vi "nanocal -- generate 3D curvature ellipsoid --  V4.vi"(6 "sampling vicinity size (%)":dbl, 7 "error mode":T7=enum."errors-linear", 8 "newton parameters":T9={"newton action"=enum."onlygrads", "weighting"=enum."dω √(|dz/dω|)", "PID-P"=0.009761510697263134, "PID-I"=5} {"PID-P" scale=1e-09..1.0 scale format="%#_3p"}, 9 "data":T8={"dz/dω  (sec/rad)"=[], "z "=[1.7183506006211996e-05-0.0001154032788780638i, 1.7124360968751133e-05-0.0001154114779288915i, 1.7049104347380084e-05-0.00011541542942613611i, 1.700437896335042e-05-0.00011541749156201827i, 1.6984579723285106e-05-0.00011542204741013496i, 1.702277369054923e-05-0.00011543195548892015i, 1.713094025845651e-05-0.00011543928112855599i, 1.734249707866828e-05-0.00011543960094139092i, 1.768320429215342e-05-0.0001154245402225022i, 1.8195281152538477e-05-0.00011538335923575508i, 1.8917228661806973e-05-0.00011530288392402138i, 1.9897834564883332e-05-0.00011516640933089982i, 2.154104046962704e-05-0.0001148906117047364i, 2.3247799321765792e-05-0.00011455940834964969i, 2.5364678450551808e-05-0.00011410149936074356i, 2.8645788781885885e-05-0.00011331572480450341i, 3.204749554800641e-05-0.00011242961468546203i, 3.783559691555022e-05-0.00011080033368711338i, 4.245015867332296e-05-0.00010941815048749576i, 4.909131821431355e-05-0.0001073312840925185i, 5.511821898441184e-05-0.00010535829212367013i, 6.178843506022867e-05-0.00010310289174359778i, 7.1079604965352e-05-9.985157907779013e-05i, 7.922304381453334e-05-9.690255343156676e-05i, 8.814778883893872e-05-9.35627973091444e-05i, 9.806709148886077e-05-8.971246458508318e-05i, 0.00011119043245647465-8.437841897470898e-05i, 0.00012253184919712196-7.953180105990741e-05i, 0.00013777724317049346-7.26422052575784e-05i, 0.0001508081004573332-6.638511645494567e-05i, 0.00016547294918783876-5.890291826790314e-05i, 0.00018003847596605868-5.097295421607585e-05i, 0.00019518361086534857-4.2160672625888326e-05i, 0.00021134179818259658-3.207632261667366e-05i, 0.0002372041782935464-1.434566976209705e-05i, 0.00025518143132024254-7.65423157605567e-07i, 0.0002835129702467886+2.297908707067173e-05i, 0.0003060118087631287+4.414715126576145e-05i, 0.00032860772064336976+6.780161699354136e-05i, 0.0003492674091322389+9.188627597766353e-05i, 0.00037498324855458583+0.0001258445655672888i, 0.00040021078021115026+0.00016463936720210011i, 0.00041969942568205823+0.0001996255883353531i, 0.00044367338947118773+0.00025154867300893595i, 0.0004634793607238068+0.0003068834938295352i, 0.00047921028781215815+0.00036805191402776324i, 0.0004880906353641744+0.00042166295770603194i, 0.0004932212623741357+0.0004947057496862386i, 0.000491476456593048+0.0005562791342814882i, 0.000480893803992059+0.0006363872629062725i, 0.0004535995818650303+0.0007373086546111893i, 0.000417087772881063+0.0008226852134031236i, 0.0003564148692854789+0.0009214817173403453i, 0.0003049201646356487+0.0009841224100520793i, 0.00021260191240459413+0.0010684135492785532i, 0.00011714858948470126+0.001130293664798013i, 1.675457544365132e-05+0.0011752384955043165i, -6.8674075405897e-05+0.0012001399159748158i, -0.000156473047607305+0.0012143601357779102i, -0.00026709373934749337+0.0012167952520739987i, -0.0003544271565676041+0.001206585218500233i, -0.00047937600197311275+0.0011721904461218277i, -0.0006086290582260493+0.0011080263068835828i, -0.0007031877411848573+0.0010369948237613604i, -0.0007564526901441745+0.0009845652865779295i, -0.000802489180995596+0.0009292050493656664i, -0.0008414596018105983+0.0008721985101652608i, -0.0008809346482248761+0.0008000538120167723i, -0.0009073902840241921+0.0007382113118499092i, -0.0009264953054508651+0.000680980624166274i, -0.0009405659412141811+0.0006247883223244968i, -0.000951649722530156+0.0005564170049287236i, -0.0009557485581057351+0.0005027508202624884i, -0.0009558464741053665+0.0004515634249715623i, -0.0009509110176922098+0.0003899637122391104i, -0.0009411315169847015+0.00033238768338539245i, -0.0009303400913929496+0.0002890952314710416i, -0.0009171113529290538+0.00024772942260094455i, -0.0009022111527275027+0.00020961974320628598i, -0.0008813746494947608+0.00016554205395646727i, -0.0008581837971946129+0.00012481593212717478i, -0.0008372063466683705+9.328565348151487e-05i, -0.0008165626610594428+6.595676342721183e-05i, -0.0007901155435838691+3.51376371228606e-05i, -0.0007682834352800848+1.2585785624721776e-05i, -0.000746231015527196-7.956667433689733e-06i, -0.0007238798463130141-2.6771164006128246e-05i, -0.0007015567569177018-4.3779400880525094e-05i, -0.000679301954671598-5.9154880569231366e-05i, -0.0006572001413831251-7.301304884663801e-05i, -0.000629855254567978-8.838260380910578e-05i, -0.0006083942229188815-9.917719243438264e-05i, -0.0005768631156754208-0.00011317657292622015i, -0.0005562177438951648-0.00012121832857134644i, -0.0005359092039599222-0.00012831021292074535i, -0.0005145186443378148-0.00013494179211461784i, -0.0004951602053444319-0.00014023403510992087i, -0.00047624970229075174-0.00014478034103386663i, -0.0004577401041527736-0.00014865456703421655i, -0.00043519037796120065-0.00015262867452433312i], "ω (rad/sec)"=[32012.991918577427, 32390.261658505893, 32466.39798177853, 32499.14340521798, 32517.39286113775, 32529.046092051318, 32537.14525712326, 32543.111142615544, 32547.696343954158, 32551.33675949651, 32554.302325209504, 32556.769142360055, 32558.856995237307, 32560.650202739795, 32562.209843476354, 32563.58125099723, 32564.7987833122, 32565.88895894197, 32566.872575330308, 32567.766175404246, 32568.583086316496, 32569.334166794306, 32570.02835688638, 32570.673085530187, 32571.274580490695, 32571.838104118455, 32572.36813539066, 32572.868514009202, 32573.342552524307, 32573.793126289274, 32574.222746575288, 32574.633618125405, 32575.027687968828, 32575.40668442971, 32575.772149741057, 32576.12546690325, 32576.467883345118, 32576.800529469096, 32577.124435064776, 32577.440543590797, 32577.749724325146, 32578.052781957467, 32578.35046682089, 32578.643482565894, 32578.932492128843, 32579.218126471686, 32579.500987779396, 32579.781656707495, 32580.06069600583, 32580.338656060805, 32580.616078519142, 32580.89350097748, 32581.171461032456, 32581.45050033079, 32581.73116925889, 32582.0140305666, 32582.29966469628, 32582.58867447239, 32582.88169000423, 32583.179375080817, 32583.48243271314, 32583.791613234323, 32584.10772197351, 32584.43162756919, 32584.764273480003, 32585.106690135035, 32585.460007297228, 32585.825472395412, 32586.204468856296, 32586.59853891288, 32587.009410462997, 32587.439030535847, 32587.889604513977, 32588.363642815923, 32588.86402143446, 32589.39405291983, 32589.957576334426, 32590.559071508098, 32591.203800151903, 32591.897990030815, 32592.64907072179, 32593.46598163404, 32594.359581707977, 32595.343197883154, 32596.433373726086, 32597.650906041054, 32599.022313348767, 32600.58195429849, 32602.375161800977, 32604.46301467823, 32606.929831615616, 32609.895397541775, 32613.535812870963, 32618.12101442274, 32624.086899701866, 32632.186064986967, 32643.839295900536, 32662.088751820305, 32694.834175046595, 32770.97049853239]}, 10 "Curvature triplet array IN":T2[](array[typedef])=[{"one"=enum."τ1", "two"=enum."στ1", "sigmaone"=enum."στ1", "sigmatwo"=enum."στ1", "3D curvature"={"curvature Matrix"=[[3.0, 1.0], [1.0, 4.0]], "eigenvs"=[4.618033988749895, 2.381966011250105], "Eigenvectors"=[[-0.8506508083520399+0.0i, -0.5257311121191335+0.0i], [0.5257311121191335+0.0i, -0.8506508083520399+0.0i]], "theta (rad)"=0.5535743588970453, "theta (deg)"=31.717474411461012, "Δs"=[4.618033988749895, 2.381966011250105], "δG/G"=0.5535743588970453, "Δlog(s)"=[4.618033988749895, 2.381966011250105], "inverse Matrix"=[[3.0, 1.0], [1.0, 4.0]], "noise T"=0.5535743588970453}, "three"=enum."στ1", "sigmathree"=enum."τ1", "pars & errors"={}}] {"3D curvature"."noise T" format="%#_3f"; "3D curvature"."inverse Matrix" format="%#_3p"; "3D curvature"."Δlog(s)" scale=0.001..10.0; "3D curvature"."δG/G" format="%#_3f"; "3D curvature"."Δs" format="%#_2p"; "3D curvature"."theta (deg)" format="%#_3p"; "3D curvature"."curvature Matrix" format="%#_3p"; "3D curvature"."eigenvs" format="%#_2f"; "3D curvature"."Eigenvectors" format="%#_3p"; "3D curvature"."theta (rad)" format="%#_3p"}, 11 "parameter map":map{T3, dbl}(c390)) -> (2 "Curvature triplet array OUT":T2[](array[typedef])=[{"one"=enum."τ1", "two"=enum."στ1", "sigmaone"=enum."στ1", "sigmatwo"=enum."στ1", "3D curvature"={"curvature Matrix"=[[3.0, 1.0], [1.0, 4.0]], "eigenvs"=[4.618033988749895, 2.381966011250105], "Eigenvectors"=[[-0.8506508083520399+0.0i, -0.5257311121191335+0.0i], [0.5257311121191335+0.0i, -0.8506508083520399+0.0i]], "theta (rad)"=0.5535743588970453, "theta (deg)"=31.717474411461012, "Δs"=[4.618033988749895, 2.381966011250105], "δG/G"=0.5535743588970453, "Δlog(s)"=[4.618033988749895, 2.381966011250105], "inverse Matrix"=[[3.0, 1.0], [1.0, 4.0]], "noise T"=0.5535743588970453}, "three"=enum."στ1", "sigmathree"=enum."τ1", "pars & errors"={}}] {"3D curvature"."noise T" format="%#_3f"; "3D curvature"."inverse Matrix" format="%#_3p"; "3D curvature"."Δlog(s)" scale=0.001..10.0; "3D curvature"."δG/G" format="%#_3f"; "3D curvature"."Δs" format="%#_2p"; "3D curvature"."theta (deg)" format="%#_3p"; "3D curvature"."curvature Matrix" format="%#_3p"; "3D curvature"."eigenvs" format="%#_2f"; "3D curvature"."Eigenvectors" format="%#_3p"; "3D curvature"."theta (rad)" format="%#_3p"})   [LabVIEW 2021]
uses:
  3-lorentzian-parameters.ctl
  nanocal -- gradient descent -- parameters.ctl
  3-lorentzian-heat-response action.ctl
  nanocal-goodness-weighting-strategy.ctl
  nanocal -- gradient descent-- data.ctl
  nanocal generate curvature ellipse -- action.ctl
  3D curvature triplet control.ctl
  3D curvature tensor.ctl
  <vilib>/Analysis/Matrix/Datatypes/RealMatrix.ctl
  <vilib>/Analysis/Matrix/Datatypes/ComplexMatrix.ctl
  3-vec.ctl
  4-vec-array.ctl
  nanocal -- gradient descent -- action.ctl
  <vilib>/Analysis/baseanly.llb/Mean (DBL).vi
  3D curvature tensor algebra --V2.vi
  array -- bilinear regression 3D -- V3.vi
  <vilib>/Analysis/7linalg.llb/Solve Linear Equations.vi
  <vilib>/Analysis/7linalg.llb/Solve Linear Equations (single right hand).vi
  array -- linear regression 3D -- V2.vi
  <vilib>/Analysis/baseanly.llb/A x B.vi
  <vilib>/Analysis/baseanly.llb/Real A x B.vi
  <vilib>/Analysis/baseanly.llb/Solve Linear Equations By Cholesky.vi
  <vilib>/Analysis/baseanly.llb/Real Matrix to Compact Array.vi
  <vilib>/Analysis/baseanly.llb/Real Compact Tri-Matrix Linear Eqs.vi
  <vilib>/Analysis/Matrix/Numeric/Conversions/Array To Matrix.vi
  <vilib>/Analysis/Matrix/Numeric/Conversions/Array To Matrix - RA2.vi
  <vilib>/Analysis/7linalg.llb/Solve Linear Eqs (General).vi
  <vilib>/Analysis/7linalg.llb/Solve Linear Eqs (Gen, single right hand).vi
  <vilib>/Analysis/Matrix/Numeric/Conversions/Matrix To Array.vi
  <vilib>/Analysis/Matrix/Numeric/Conversions/Matrix To Array - RM.vi
  <vilib>/Analysis/7linalg.llb/Eigenvalues and Vectors.vi
  <vilib>/Analysis/7linalg.llb/Real Eigenvalues and Vectors.vi
  <vilib>/Analysis/baseanly.llb/Inverse Matrix.vi
  <vilib>/Analysis/baseanly.llb/Real Inverse Matrix.vi
  <vilib>/Analysis/NI_AALBase.lvlib
  <vilib>/Analysis/Matrix/NI_Matrix.lvlib
panel:
  in  "means":T1
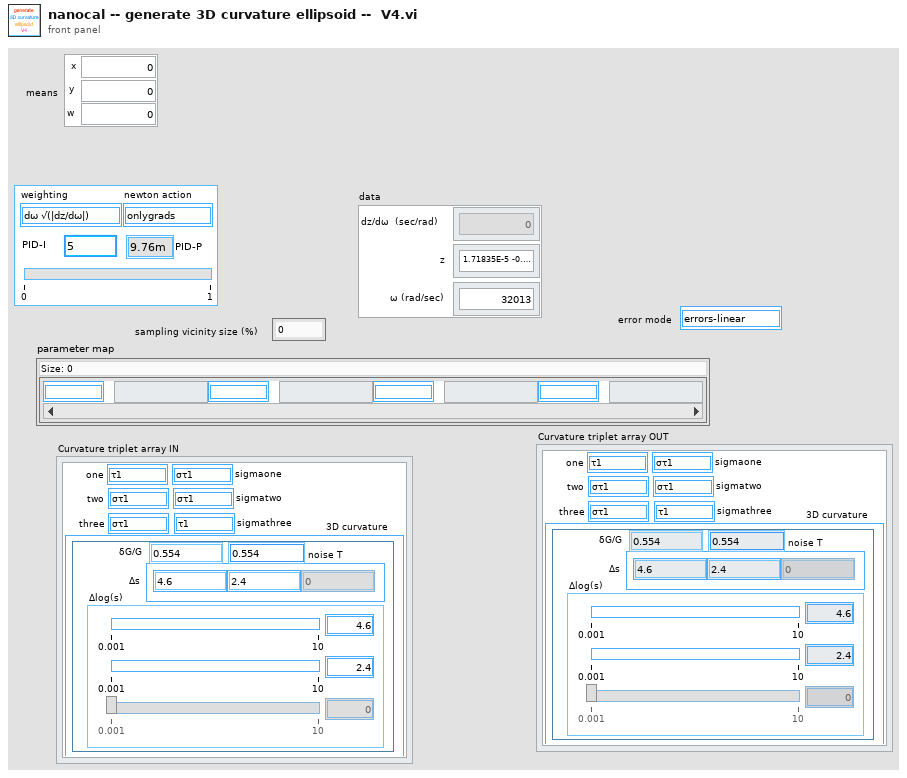
[diagram p1: front panel]
types:
  T1 = typedef "3-vec.ctl" = cluster{"x":dbl, "y":dbl, "w":dbl}
  T2 = typedef "3D curvature triplet control.ctl" = cluster{"one":T3, "two":T3, "sigmaone":T3, "sigmatwo":T3, "3D curvature":T4, "three":T3, "sigmathree":T3, "pars & errors":map{T3, dbl}}
  T3 = typedef "3-lorentzian-parameters.ctl" = enum16{"ζ", "τ1", "τS", "τN", "τC", "κ0", "m1", "m2", "m3", "T (K)", "B (T)", "θ (deg)", "side (S|R)", "set of (B|T)", "Re(offset)", "Im(offset)", "στ1", "στ1-", "στ1+", "στS", "στS-", "στS+", "στN", "στN-", "στN+"}
  T4 = typedef "3D curvature tensor.ctl" = cluster{"curvature Matrix":T5, "eigenvs":dbl[], "Eigenvectors":T6, "theta (rad)":dbl, "theta (deg)":dbl, "Δs":dbl[], "δG/G":dbl, "Δlog(s)":dbl[], "inverse Matrix":T5, "noise T":dbl}
  T5 = typedef "NI_Matrix.lvlib/RealMatrix.ctl" = dbl[][]
  T6 = typedef "NI_Matrix.lvlib/ComplexMatrix.ctl" = cdb[][]
  T7 = typedef "nanocal generate curvature ellipse -- action.ctl" = enum16{"errors-log", "errors-linear"}
  T8 = typedef "nanocal -- gradient descent-- data.ctl" = cluster{"dz/dω  (sec/rad)":cdb[], "z ":cdb[], "ω (rad/sec)":dbl[]}
  T9 = typedef "nanocal -- gradient descent -- parameters.ctl" = cluster{"newton action":T10, "weighting":T11, "PID-P":dbl, "PID-I":i32}
  T10 = typedef "3-lorentzian-heat-response action.ctl" = enum16{"calc R", "create string", "calc m1m2m3", "dζ", "dT1", "dτS", "dτN", "dτC", "d-all", "dκ0", "T(K)", "m1", "m2", "m3", "parse string", "θ (deg)", "B (T)", "onlygrads", "newton", "create emty string"}
  T11 = typedef "nanocal-goodness-weighting-strategy.ctl" = enum16{"dω", "dω √(|dz/dω|)", "dω |dz/dω|", "phase", "andreas", "sum", "1/f noise"}
  T12 = typedef "4-vec-array.ctl" = cluster{"x":dbl[], "y":dbl[], "w":dbl[], "z":dbl[]}
  T13 = typedef "nanocal -- gradient descent -- action.ctl" = enum16{"init", "step", "peek"}
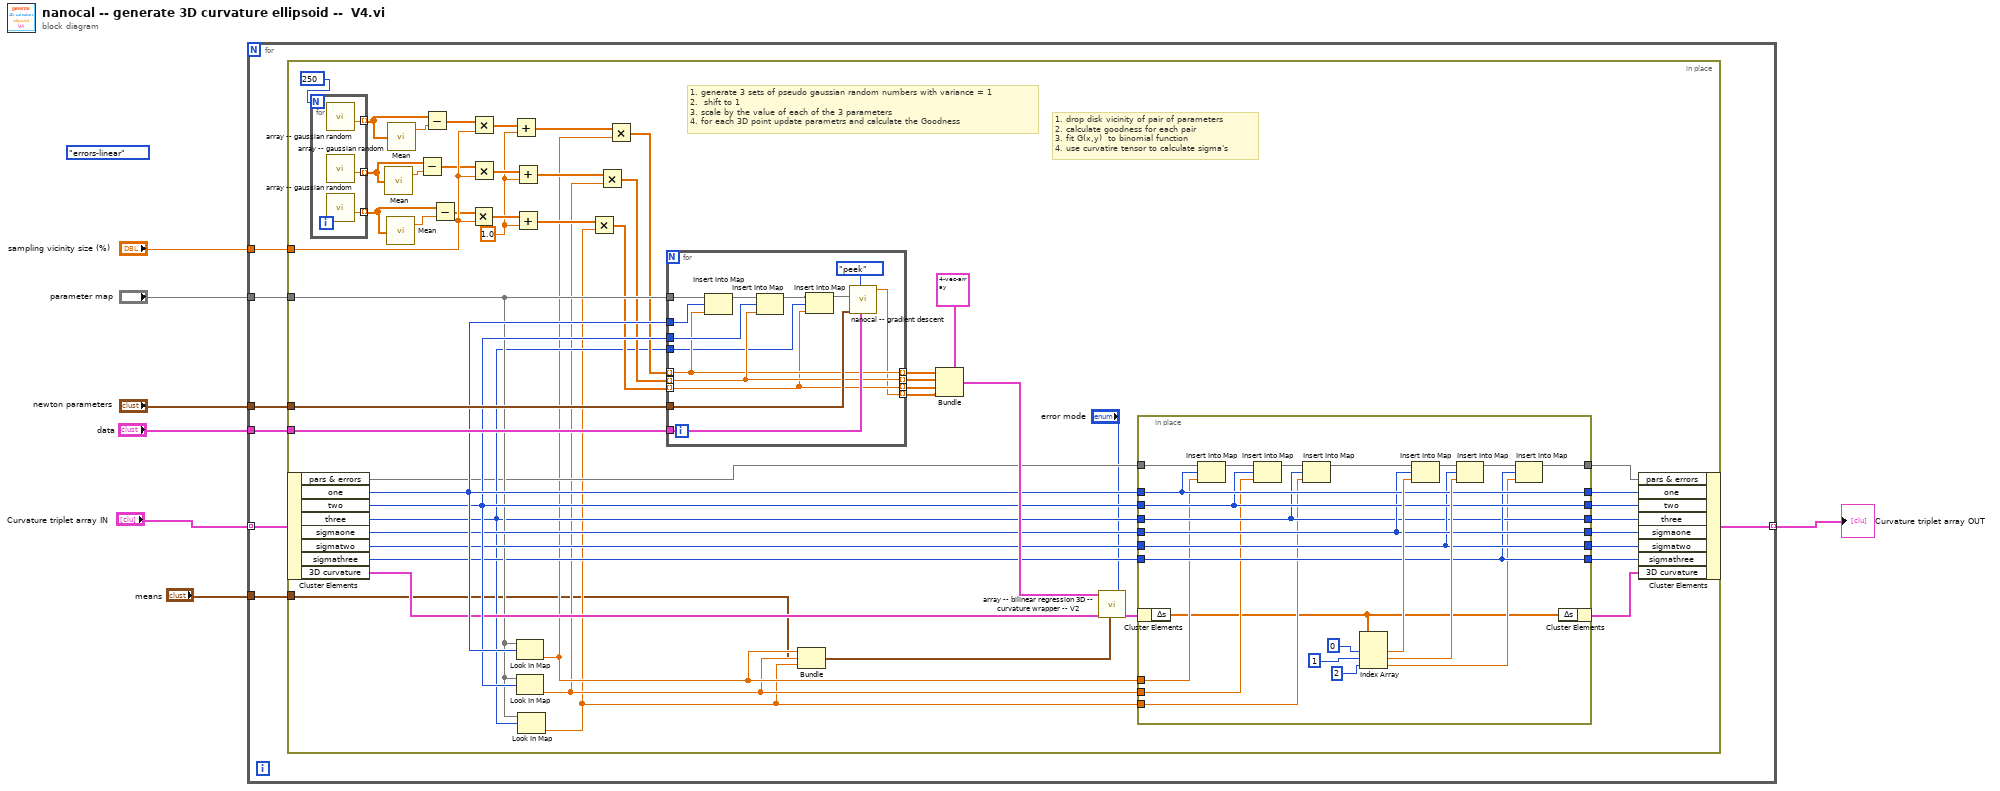
[diagram p0: block diagram]
diagram:
  (unwired) nanocal_generate_curvature_ellipse_--_action."errors-linear" ("Enum")
  n1 = for {
    tunnel: "newton parameters" -> [w14]
    tunnel: "data" -> [w13]
    tunnel: [w9] -> w2 mode=indexing
    tunnel: "sampling vicinity size (%)" -> [w12]
    tunnel: "parameter map" -> [w11]
    tunnel: "Curvature triplet array IN" -> [w10] mode=indexing
    tunnel: "means" -> [w8]
    n2 = in-place {
      in-place-border: w14 -> [w67]
      in-place-border: w13 -> [w65]
      in-place-border: w12 -> [w43]
      in-place-border: w11 -> [w54]
      in-place-border: w8 -> [w21]
      w42 = 1.0 ("number")
      # "1. generate 3 sets of pseudo gaussian random numbers with variance = 1 \n2.  shift to 1\n3. scale by the value of each of the 3 parameters \n4. for each 3D point update parametrs and calculate the Goodness"
      # "1. drop disk vicinity of pair of parameters \n2. calculate goodness for each pair \n3. fit G(x,y)  to binomial function \n4. use curvatire tensor to calculate sigma's"
      n3 = in-place-cluster #1(w10) -> ("pars & errors"=w36:map{T3, dbl}, "one"=w63:T3, "two"=w62:T3, "three"=w38:T3, "sigmaone"=w61:T3, "sigmatwo"=w60:T3, "sigmathree"=w52:T3, "3D curvature"=w55:T4)
      n4 = for {
        N: 250 -> [_]
        tunnel: [w70] -> w33 mode=indexing
        tunnel: [w69] -> w29 mode=indexing
        tunnel: [w68] -> w31 mode=indexing
        n5 = call "array -- gaussian random.vi"() -> ("number"=w70:dbl)  [unwired: 11 in]
        n6 = call "array -- gaussian random.vi"() -> ("number"=w69:dbl)  [unwired: 11 in]
        n7 = call "array -- gaussian random.vi"() -> ("number"=w68:dbl)  [unwired: 11 in]
      }
      n8 = call-poly <vilib>:"Mean.vi"("X"=w29) -> ("mean"=w27:dbl)  [unwired: 1 out]
      n9 = call-poly <vilib>:"Mean.vi"("X"=w31) -> ("mean"=w32:dbl)  [unwired: 1 out]
      n10 = call-poly <vilib>:"Mean.vi"("X"=w33) -> ("mean"=w34:dbl)  [unwired: 1 out]
      n11 = Subtract(x=w29, y=w27) -> (x-y=w28:dbl[])
      n12 = Subtract(x=w33, y=w34) -> (x-y=w35:dbl[])
      n13 = Subtract(x=w31, y=w32) -> (x-y=w30:dbl[])
      n14 = Multiply(x=w30, y=w43) -> (x*y=w45:dbl[])
      n15 = Multiply(x=w35, y=w43) -> (x*y=w49:dbl[])
      n16 = Multiply(x=w28, y=w43) -> (x*y=w47:dbl[])
      n17 = Add(x=w49, y=w42) -> (x+y=w48:dbl[])
      n18 = Add(x=w47, y=w42) -> (x+y=w46:dbl[])
      n19 = Add(x=w45, y=w42) -> (x+y=w44:dbl[])
      n20 = Look In Map(map=w54, key=w63) -> (value=w25:dbl)  [unwired: 1 in, 1 out]
      n21 = Look In Map(map=w54, key=w62) -> (value=w24:dbl)  [unwired: 1 in, 1 out]
      n22 = Look In Map(map=w54, key=w38) -> (value=w23:dbl)  [unwired: 1 in, 1 out]
      n23 = Multiply(x=w44, y=w23) -> (x*y=w39:dbl[])
      n24 = Multiply(x=w46, y=w24) -> (x*y=w40:dbl[])
      n25 = Multiply(x=w48, y=w25) -> (x*y=w41:dbl[])
      n26 = for {
        tunnel: w63 -> [w102]
        tunnel: w62 -> [w106]
        tunnel: w41 -> [w99] mode=indexing
        tunnel: w40 -> [w100] mode=indexing
        tunnel: w67 -> [w104]
        tunnel: w54 -> [w103]
        tunnel: [w95] -> w18 mode=indexing
        tunnel: w65 -> [w101]
        tunnel: [w100] -> w19 mode=indexing
        tunnel: [w99] -> w20 mode=indexing
        tunnel: w39 -> [w95] mode=indexing
        tunnel: w38 -> [w96]
        tunnel: [w94] -> w17 mode=indexing
        n27 = Insert Into Map(map in=w103, key=w102, value=w99) -> (map out=w107:map{T3, dbl})  [unwired: 2 out]
        n28 = Insert Into Map(map in=w107, key=w106, value=w100) -> (map out=w98:map{T3, dbl})  [unwired: 2 out]
        n29 = Insert Into Map(map in=w98, key=w96, value=w95) -> (map out=w97:map{T3, dbl})  [unwired: 2 out]
        n30 = call "nanocal -- gradient descent.vi"("data"=w101, "action"=nanocal_--_gradient_descent_--_action."peek", "newton pars"=w104, "parameter Map IN"=w97) -> ("goodness OUT"=w94:dbl)  [unwired: 3 in, 4 out]
      }
      n31 = Bundle(cluster=w21, "x"=w25, "y"=w24, "w"=w23) -> (w22:T1)
      n32 = Bundle(cluster=T12 {"x"=[-2.0, -1.0, 0.0, 1.0, 2.0], "y"=[-2.0, -1.0, 0.0, 1.0, 2.0], "w"=[-2.0, -1.0, 0.0, 1.0, 2.0], "z"=[12.0, 3.0, 0.0, 3.0, 12.0]} ("xyzw  IN"), "x"=w20, "y"=w19, "w"=w18, "z"=w17) -> (w66:T12)
      n33 = call "array -- bilinear regression 3D -- curvature wrapper -- V2.vi"("error mode"="error mode", "means"=w22, "3D curvature tensor IN"=w55, "xyzw  IN"=w66) -> ("3D curvature tensor OUT"=w26:T4)  [unwired: 5 in, 2 out]
      n34 = in-place {
        in-place-border: w25 -> [w74]
        in-place-border: w24 -> [w73]
        in-place-border: w63 -> [w87]
        in-place-border: w62 -> [w86]
        in-place-border: w61 -> [w85]
        in-place-border: w60 -> [w84]
        in-place-border: [w87] -> w59
        in-place-border: [w86] -> w58
        in-place-border: [w85] -> w57
        in-place-border: [w84] -> w56
        in-place-border: w36 -> [w82]
        in-place-border: [w78] -> w37
        in-place-border: w23 -> [w72]
        in-place-border: [w77] -> w53
        in-place-border: w52 -> [w77]
        in-place-border: w38 -> [w76]
        in-place-border: [w76] -> w51
        n35 = in-place-cluster #2(w26) -> ("Δs"=w71:dbl[])
        n36 = Insert Into Map(map in=w82, key=w87, value=w74) -> (map out=w88:map{T3, dbl})  [unwired: 2 out]
        n37 = Insert Into Map(map in=w88, key=w86, value=w73) -> (map out=w81:map{T3, dbl})  [unwired: 2 out]
        n38 = Insert Into Map(map in=w81, key=w76, value=w72) -> (map out=w80:map{T3, dbl})  [unwired: 2 out]
        n39 = Index Array(array=w71, index #1=0 ("index"), index #2=1 ("index"), index #3=2 ("index")) -> (element #1=w92:dbl, element #2=w93:dbl, element #3=w75:dbl)
        n40 = Insert Into Map(map in=w80, key=w85, value=w92) -> (map out=w91:map{T3, dbl})  [unwired: 2 out]
        n41 = Insert Into Map(map in=w91, key=w84, value=w93) -> (map out=w79:map{T3, dbl})  [unwired: 2 out]
        n42 = Insert Into Map(map in=w79, key=w77, value=w75) -> (map out=w78:map{T3, dbl})  [unwired: 2 out]
        n43 = in-place-cluster #2("Δs"=w71) -> (w64:T4)
      }
      n44 = in-place-cluster #1("pars & errors"=w37, "one"=w59, "two"=w58, "three"=w51, "sigmaone"=w57, "sigmatwo"=w56, "sigmathree"=w53, "3D curvature"=w64) -> (w9:T2)
    }
  }
  "Curvature triplet array OUT" <- w2
